vi "Rotate CCW.vi"(10 "Direction":T1) -> (2 "CCW Rotated":T1)   [LabVIEW 2020, in "SquareBattle.lvlib"]
doc: "Given a direction, this VI returns the direction that is 45 degrees rotated counter-clockwise. E.g. if N is specified, the returned value will be NW and if W is specified SW will be returned."
uses:
  SquareBattle.lvlib
  Direction.ctl
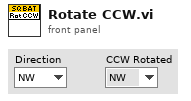
[diagram p1: front panel]
types:
  T1 = typedef "SquareBattle.lvlib/Direction.ctl" = enum16{"NW", "N", "NE", "E", "SE", "S", "SW", "W"}
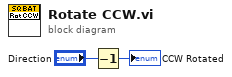
[diagram p0: block diagram]
diagram:
  n1 = Decrement(x="Direction") -> (x-1=→"CCW Rotated":T1)
